vi "rsidr_core_global.vi"() -> ()   [LabVIEW 2020, in "Rohde&Schwarz CMWXP NR FR1 Measurement.lvlib"] (continued)
count for modulation measurements exceeding the specified modulation limits.\nDefault unit:  %\n\n<3_Ripple1>\n float\nMax (range 1) - min (range 1)\nDefault unit:  dB\n\n<4_Ripple2>\n float\nMax (range 2) - min (range 2)\nDefault unit:  dB\n\n<5_MaxR1MinR2>\n float\nMax (range 1) - min (range 2)\nDefault unit:  dB\n\n<6_MaxR2MinR1>\n float\nMax (range 2) - min (range 1)\nDefault unit:  dB\n\n<7_MinR1>\n float\nMin (range 1)\nDefault unit:  dB\n\n<8_MaxR1>\n float\nMax (range 1)\nDefault unit:  dB\n\n<9_MinR2>\n float\nMin (range 2)\nDefault unit:  dB\n\n<10_MaxR2>\n float\nMax (range 2)\nDefault unit:  dB\n\nAvailable Repeated Capabilities:\ninstance: i0, i1, i2, i3, i4, i5, i6, i7, i8, i9, i10, i11, i12, i13, i14, i15, i16, i17, i18, i19, i20, i21, i22, i23, i24, i25, i26, i27, i28, i29, i30, i31, i32\r\n\nRemote-control command(s):\nREAD:NRSub:MEAS<i>:MEValuation:ESFLatness:EXTReme?"}, {"Level"=4, "Class Only"=FALSE, "Identifier"="RSCMWXPNRFR1M_ATTR_READ_MULTI_EVAL_MEAS_ES_FLATNESS_STANDARD_DEVIATION_RESULTS", "Descriptive Name"="Read Multi Eval Meas ES Flatness Standard Deviation Results", "Data Type"=enum."RawString", "Command"="READ:NRS:MEAS{instance}:MEV:ESFL:SDEV?", "Access"=enum."Read Only", "Range Table"="", "Read Callback"="", "Write Callback"="", "Range Callback"="", "Check Callback"="", "Rngtable Callback"="", "Coerce Callback"="", "Supported Models"="", "Instrument Options"="", "Check Status Callback"="", "Flags"=0, "Help"="Return standard deviation single value results of the equalizer spectrum flatness measurement.\n\n<1_Reliability>\n decimal\n\n<2_OutOfTol>\n decimal\nOut of tolerance result, i.e. percentage of measurement intervals of the statistic count for modulation measurements exceeding the specified modulation limits.\nDefault unit:  %\n\n<3_Ripple1>\n float\nMax (range 1) - min (range 1)\nDefault unit:  dB\n\n<4_Ripple2>\n float\nMax (range 2) - min (range 2)\nDefault unit:  dB\n\n<5_MaxR1MinR2>\n float\nMax (range 1) - min (range 2)\nDefault unit:  dB\n\n<6_MaxR2MinR1>\n float\nMax (range 2) - min (range 1)\nDefault unit:  dB\n\n<7_MinR1>\n float\nMin (range 1)\nDefault unit:  dB\n\n<8_MaxR1>\n float\nMax (range 1)\nDefault unit:  dB\n\n<9_MinR2>\n float\nMin (range 2)\nDefault unit:  dB\n\n<10_MaxR2>\n float\nMax (range 2)\nDefault unit:  dB\n\nAvailable Repeated Capabilities:\ninstance: i0, i1, i2, i3, i4, i5, i6, i7, i8, i9, i10, i11, i12, i13, i14, i15, i16, i17, i18, i19, i20, i21, i22, i23, i24, i25, i26, i27, i28, i29, i30, i31, i32\r\n\nRemote-control command(s):\nREAD:NRSub:MEAS<i>:MEValuation:ESFLatness:SDEViation?"}, {"Level"=4, "Class Only"=FALSE, "Identifier"="RSCMWXPNRFR1M_ATTR_FETCH_MULTI_EVAL_MEAS_ES_FLATNESS_CURRENT_RESULTS", "Descriptive Name"="Fetch Multi Eval Meas ES Flatness Current Results", "Data Type"=enum."RawString", "Command"="FETC:NRS:MEAS{instance}:MEV:ESFL:CURR?", "Access"=enum."Read Only", "Range Table"="", "Read Callback"="", "Write Callback"="", "Range Callback"="", "Check Callback"="", "Rngtable Callback"="", "Coerce Callback"="", "Supported Models"="", "Instrument Options"="", "Check Status Callback"="", "Flags"=0, "Help"="Return current single value results of the equalizer spectrum flatness measurement.\n\n<1_Reliability>\n decimal\n\n<2_OutOfTol>\n decimal\nOut of tolerance result, i.e. percentage of measurement intervals of the statistic count for modulation measurements exceeding the specified modulation limits.\nDefault unit:  %\n\n<3_Ripple1>\n float\nMax (range 1) - min (range 1)\nDefault unit:  dB\n\n<4_Ripple2>\n float\nMax (range 2) - min (range 2)\nDefault unit:  dB\n\n<5_MaxR1MinR2>\n float\nMax (range 1) - min (range 2)\nDefault unit:  dB\n\n<6_MaxR2MinR1>\n float\nMax (range 2) - min (range 1)\nDefault unit:  dB\n\n<7_MinR1>\n float\nMin (range 1)\nDefault unit:  dB\n\n<8_MaxR1>\n float\nMax (range 1)\nDefault unit:  dB\n\n<9_MinR2>\n float\nMin (range 2)\nDefault unit:  dB\n\n<10_MaxR2>\n float\nMax (range 2)\nDefault unit:  dB\n\nAvailable Repeated Capabilities:\ninstance: i0, i1, i2, i3, i4, i5, i6, i7, i8, i9, i10, i11, i12, i13, i14, i15, i16, i17, i18, i19, i20, i21, i22, i23, i24, i25, i26, i27, i28, i29, i30, i31, i32\r\n\nRemote-control command(s):\nFETCh:NRSub:MEAS<i>:MEValuation:ESFLatness:CURRent?"}, {"Level"=4, "Class Only"=FALSE, "Identifier"="RSCMWXPNRFR1M_ATTR_FETCH_MULTI_EVAL_MEAS_ES_FLATNESS_AVERAGE_RESULTS", "Descriptive Name"="Fetch Multi Eval Meas ES Flatness Average Results", "Data Type"=enum."RawString", "Command"="FETC:NRS:MEAS{instance}:MEV:ESFL:AVER?", "Access"=enum."Read Only", "Range Table"="", "Read Callback"="", "Write Callback"="", "Range Callback"="", "Check Callback"="", "Rngtable Callback"="", "Coerce Callback"="", "Supported Models"="", "Instrument Options"="", "Check Status Callback"="", "Flags"=0, "Help"="Return average single value results of the equalizer spectrum flatness measurement.\n\n<1_Reliability>\n decimal\n\n<2_OutOfTol>\n decimal\nOut of tolerance result, i.e. percentage of measurement intervals of the statistic count for modulation measurements exceeding the specified modulation limits.\nDefault unit:  %\n\n<3_Ripple1>\n float\nMax (range 1) - min (range 1)\nDefault unit:  dB\n\n<4_Ripple2>\n float\nMax (range 2) - min (range 2)\nDefault unit:  dB\n\n<5_MaxR1MinR2>\n float\nMax (range 1) - min (range 2)\nDefault unit:  dB\n\n<6_MaxR2MinR1>\n float\nMax (range 2) - min (range 1)\nDefault unit:  dB\n\n<7_MinR1>\n float\nMin (range 1)\nDefault unit:  dB\n\n<8_MaxR1>\n float\nMax (range 1)\nDefault unit:  dB\n\n<9_MinR2>\n float\nMin (range 2)\nDefault unit:  dB\n\n<10_MaxR2>\n float\nMax (range 2)\nDefault unit:  dB\n\nAvailable Repeated Capabilities:\ninstance: i0, i1, i2, i3, i4, i5, i6, i7, i8, i9, i10, i11, i12, i13, i14, i15, i16, i17, i18, i19, i20, i21, i22, i23, i24, i25, i26, i27, i28, i29, i30, i31, i32\r\n\nRemote-control command(s):\nFETCh:NRSub:MEAS<i>:MEValuation:ESFLatness:AVERage?"}, {"Level"=4, "Class Only"=FALSE, "Identifier"="RSCMWXPNRFR1M_ATTR_FETCH_MULTI_EVAL_MEAS_ES_FLATNESS_EXTREME_RESULTS", "Descriptive Name"="Fetch Multi Eval Meas ES Flatness Extreme Results", "Data Type"=enum."RawString", "Command"="FETC:NRS:MEAS{instance}:MEV:ESFL:EXTR?", "Access"=enum."Read Only", "Range Table"="", "Read Callback"="", "Write Callback"="", "Range Callback"="", "Check Callback"="", "Rngtable Callback"="", "Coerce Callback"="", "Supported Models"="", "Instrument Options"="", "Check Status Callback"="", "Flags"=0, "Help"="Return extreme single value results of the equalizer spectrum flatness measurement.\n\n<1_Reliability>\n decimal\n\n<2_OutOfTol>\n decimal\nOut of tolerance result, i.e. percentage of measurement intervals of the statistic count for modulation measurements exceeding the specified modulation limits.\nDefault unit:  %\n\n<3_Ripple1>\n float\nMax (range 1) - min (range 1)\nDefault unit:  dB\n\n<4_Ripple2>\n float\nMax (range 2) - min (range 2)\nDefault unit:  dB\n\n<5_MaxR1MinR2>\n float\nMax (range 1) - min (range 2)\nDefault unit:  dB\n\n<6_MaxR2MinR1>\n float\nMax (range 2) - min (range 1)\nDefault unit:  dB\n\n<7_MinR1>\n float\nMin (range 1)\nDefault unit:  dB\n\n<8_MaxR1>\n float\nMax (range 1)\nDefault unit:  dB\n\n<9_MinR2>\n float\nMin (range 2)\nDefault unit:  dB\n\n<10_MaxR2>\n float\nMax (range 2)\nDefault unit:  dB\n\nAvailable Repeated Capabilities:\ninstance: i0, i1, i2, i3, i4, i5, i6, i7, i8, i9, i10, i11, i12, i13, i14, i15, i16, i17, i18, i19, i20, i21, i22, i23, i24, i25, i26, i27, i28, i29, i30, i31, i32\r\n\nRemote-control command(s):\nFETCh:NRSub:MEAS<i>:MEValuation:ESFLatness:EXTReme?"}, {"Level"=4, "Class Only"=FALSE, "Identifier"="RSCMWXPNRFR1M_ATTR_FETCH_MULTI_EVAL_MEAS_ES_FLATNESS_STANDARD_DEVIATION_RESULTS", "Descriptive Name"="Fetch Multi Eval Meas ES Flatness Standard Deviation Results", "Data Type"=enum."RawString", "Command"="FETC:NRS:MEAS{instance}:MEV:ESFL:SDEV?", "Access"=enum."Read Only", "Range Table"="", "Read Callback"="", "Write Callback"="", "Range Callback"="", "Check Callback"="", "Rngtable Callback"="", "Coerce Callback"="", "Supported Models"="", "Instrument Options"="", "Check Status Callback"="", "Flags"=0, "Help"="Return standard deviation single value results of the equalizer spectrum flatness measurement.\n\n<1_Reliability>\n decimal\n\n<2_OutOfTol>\n decimal\nOut of tolerance result, i.e. percentage of measurement intervals of the statistic count for modulation measurements exceeding the specified modulation limits.\nDefault unit:  %\n\n<3_Ripple1>\n float\nMax (range 1) - min (range 1)\nDefault unit:  dB\n\n<4_Ripple2>\n float\nMax (range 2) - min (range 2)\nDefault unit:  dB\n\n<5_MaxR1MinR2>\n float\nMax (range 1) - min (range 2)\nDefault unit:  dB\n\n<6_MaxR2MinR1>\n float\nMax (range 2) - min (range 1)\nDefault unit:  dB\n\n<7_MinR1>\n float\nMin (range 1)\nDefault unit:  dB\n\n<8_MaxR1>\n float\nMax (range 1)\nDefault unit:  dB\n\n<9_MinR2>\n float\nMin (range 2)\nDefault unit:  dB\n\n<10_MaxR2>\n float\nMax (range 2)\nDefault unit:  dB\n\nAvailable Repeated Capabilities:\ninstance: i0, i1, i2, i3, i4, i5, i6, i7, i8, i9, i10, i11, i12, i13, i14, i15, i16, i17, i18, i19, i20, i21, i22, i23, i24, i25, i26, i27, i28, i29, i30, i31, i32\r\n\nRemote-control command(s):\nFETCh:NRSub:MEAS<i>:MEValuation:ESFLatness:SDEViation?"}, {"Level"=4, "Class Only"=FALSE, "Identifier"="RSCMWXPNRFR1M_ATTR_QUERY_MULTI_EVAL_MEAS_ES_FLATNESS_CURRENT_LIMIT_CHECK_RESULTS", "Descriptive Name"="Query Multi Eval Meas ES Flatness Current Limit Check Results", "Data Type"=enum."RawString", "Command"="CALC:NRS:MEAS{instance}:MEV:ESFL:CURR?", "Access"=enum."Read Only", "Range Table"="", "Read Callback"="", "Write Callback"="", "Range Callback"="", "Check Callback"="", "Rngtable Callback"="", "Coerce Callback"="", "Supported Models"="", "Instrument Options"="", "Check Status Callback"="", "Flags"=0, "Help"="Return current limit check results for the equalizer spectrum flatness measurement.\n\nReturn values:\n<Reliability>\n decimal\n\n<OutOfTolerance>\n decimal\nOut of tolerance result, i.e. percentage of measurement intervals of the statistic count for modulation measurements exceeding the specified modulation limits.\nDefault unit:  %\n\n<Ripple1>\n Limit check result for max (range 1) - min (range 1)\n\n<Ripple2>\n Limit check result for max (range 2) - min (range 2)\n\n<MaxR1MinR2>\n Limit check result for max (range 1) - min (range 2)\n\n<MaxR2MinR1>\n Limit check result for max (range 2) - min (range 1)\n\nAvailable Repeated Capabilities:\ninstance: i0, i1, i2, i3, i4, i5, i6, i7, i8, i9, i10, i11, i12, i13, i14, i15, i16, i17, i18, i19, i20, i21, i22, i23, i24, i25, i26, i27, i28, i29, i30, i31, i32\r\n\nRemote-control command(s):\nCALCulate:NRSub:MEAS<i>:MEValuation:ESFLatness:CURRent?"}, {"Level"=4, "Class Only"=FALSE, "Identifier"="RSCMWXPNRFR1M_ATTR_QUERY_MULTI_EVAL_MEAS_ES_FLATNESS_AVERAGE_LIMIT_CHECK_RESULTS", "Descriptive Name"="Query Multi Eval Meas ES Flatness Average Limit Check Results", "Data Type"=enum."RawString", "Command"="CALC:NRS:MEAS{instance}:MEV:ESFL:AVER?", "Access"=enum."Read Only", "Range Table"="", "Read Callback"="", "Write Callback"="", "Range Callback"="", "Check Callback"="", "Rngtable Callback"="", "Coerce Callback"="", "Supported Models"="", "Instrument Options"="", "Check Status Callback"="", "Flags"=0, "Help"="Return average results for the equalizer spectrum flatness measurement.\n\nReturn values:\n<Reliability>\n decimal\n\n<OutOfTolerance>\n decimal\nOut of tolerance result, i.e. percentage of measurement intervals of the statistic count for modulation measurements exceeding the specified modulation limits.\nDefault unit:  %\n\n<Ripple1>\n Limit check result for max (range 1) - min (range 1)\n\n<Ripple2>\n Limit check result for max (range 2) - min (range 2)\n\n<MaxR1MinR2>\n Limit check result for max (range 1) - min (range 2)\n\n<MaxR2MinR1>\n Limit check result for max (range 2) - min (range 1)\n\nAvailable Repeated Capabilities:\ninstance: i0, i1, i2, i3, i4, i5, i6, i7, i8, i9, i10, i11, i12, i13, i14, i15, i16, i17, i18, i19, i20, i21, i22, i23, i24, i25, i26, i27, i28, i29, i30, i31, i32\r\n\nRemote-control command(s):\nCALCulate:NRSub:MEAS<i>:MEValuation:ESFLatness:AVERage?"}, {"Level"=4, "Class Only"=FALSE, "Identifier"="RSCMWXPNRFR1M_ATTR_QUERY_MULTI_EVAL_MEAS_ES_FLATNESS_EXTREME_LIMIT_CHECK_RESULTS", "Descriptive Name"="Query Multi Eval Meas ES Flatness Extreme Limit Check Results", "Data Type"=enum."RawString", "Command"="CALC:NRS:MEAS{instance}:MEV:ESFL:EXTR?", "Access"=enum."Read Only", "Range Table"="", "Read Callback"="", "Write Callback"="", "Range Callback"="", "Check Callback"="", "Rngtable Callback"="", "Coerce Callback"="", "Supported Models"="", "Instrument Options"="", "Check Status Callback"="", "Flags"=0, "Help"="Return extreme limit check results for the equalizer spectrum flatness measurement.\n\nReturn values:\n<Reliability>\n decimal\n\n<OutOfTolerance>\n decimal\nOut of tolerance result, i.e. percentage of measurement intervals of the statistic count for modulation measurements exceeding the specified modulation limits.\nDefault unit:  %\n\n<Ripple1>\n Limit check result for max (range 1) - min (range 1)\n\n<Ripple2>\n Limit check result for max (range 2) - min (range 2)\n\n<MaxR1MinR2>\n Limit check result for max (range 1) - min (range 2)\n\n<MaxR2MinR1>\n Limit check result for max (range 2) - min (range 1)\n\nAvailable Repeated Capabilities:\ninstance: i0, i1, i2, i3, i4, i5, i6, i7, i8, i9, i10, i11, i12, i13, i14, i15, i16, i17, i18, i19, i20, i21, i22, i23, i24, i25, i26, i27, i28, i29, i30, i31, i32\r\n\nRemote-control command(s):\nCALCulate:NRSub:MEAS<i>:MEValuation:ESFLatness:EXTReme?"}, {"Level"=4, "Class Only"=FALSE, "Identifier"="RSCMWXPNRFR1M_ATTR_FETCH_MULTI_EVAL_MEAS_ES_FLATNESS_SUBCARRIER_INDEX_RESULTS", "Descriptive Name"="Fetch Multi Eval Meas ES Flatness Subcarrier Index Results", "Data Type"=enum."RawString", "Command"="FETC:NRS:MEAS{instance}:MEV:ESFL:CURR:SCIN?", "Access"=enum."Read Only", "Range Table"="", "Read Callback"="", "Write Callback"="", "Range Callback"="", "Check Callback"="", "Rngtable Callback"="", "Coerce Callback"="", "Supported Models"="", "Instrument Options"="", "Check Status Callback"="", "Flags"=0, "Help"="Returns subcarrier indices of the equalizer spectrum flatness measurement. At these SC indices, the current minimum and maximum power of the equalizer coefficients have been detected within range 1 and range 2.\n\nReturn values:\n<Reliability>\n decimal\n\n<OutOfTolerance>\n decimal\nOut of tolerance result, i.e. percentage of measurement intervals of the statistic count for modulation measurements exceeding the specified modulation limits.\nDefault unit:  %\n\n<Maximum1>\n decimal\nSC index of 'Max (Range 1)'\n\n<Minimum1>\n decimal\nSC index of 'Min (Range 1)'\n\n<Maximum2>\n decimal\nSC index of 'Max (Range 2)'\n\n<Minimum2>\n decimal\nSC index of 'Min (Range 2)'\n\nAvailable Repeated Capabilities:\ninstance: i0, i1, i2, i3, i4, i5, i6, i7, i8, i9, i10, i11, i12, i13, i14, i15, i16, i17, i18, i19, i20, i21, i22, i23, i24, i25, i26, i27, i28, i29, i30, i31, i32\r\n\nRemote-control command(s):\nFETCh:NRSub:MEAS<i>:MEValuation:ESFLatness:CURRent:SCINdex?"}, {"Level"=3, "Class Only"=TRUE, "Identifier"="", "Descriptive Name"="Spectrum Emission Mask", "Data Type"=enum."ViInt32", "Command"="", "Access"=enum."Read Only", "Range Table"="", "Read Callback"="", "Write Callback"="", "Range Callback"="", "Check Callback"="", "Rngtable Callback"="", "Coerce Callback"="", "Supported Models"="", "Instrument Options"="", "Check Status Callback"="", "Flags"=0, "Help"="The commands in this class return the spectrum emission results."}, {"Level"=4, "Class Only"=FALSE, "Identifier"="RSCMWXPNRFR1M_ATTR_READ_MULTI_EVAL_MEAS_SEM_CURRENT_RESULTS", "Descriptive Name"="Read Multi Eval Meas SEM Current Results", "Data Type"=enum."RawString", "Command"="READ:NRS:MEAS{instance}:MEV:SEM:CURR?", "Access"=enum."Read Only", "Range Table"="", "Read Callback"="", "Write Callback"="", "Range Callback"="", "Check Callback"="", "Rngtable Callback"="", "Coerce Callback"="", "Supported Models"="", "Instrument Options"="", "Check Status Callback"="", "Flags"=0, "Help"="Return the current single value results of the spectrum emission measurement.\n\nReturn values:\n<Reliability>\n decimal\n\n<OutOfTolerance>\n decimal\nOut of tolerance result, i.e. percentage of measurement intervals of the statistic count for spectrum emission measurements exceeding the specified spectrum emission mask limits.\nDefault unit:  % \n\n<OBW>\n float\nOccupied bandwidth\nDefault unit:  Hz \n\n<TXpower>\n float\nTotal TX power in the slot\nDefault unit:  dBm\n\nAvailable Repeated Capabilities:\ninstance: i0, i1, i2, i3, i4, i5, i6, i7, i8, i9, i10, i11, i12, i13, i14, i15, i16, i17, i18, i19, i20, i21, i22, i23, i24, i25, i26, i27, i28, i29, i30, i31, i32\r\n\nRemote-control command(s):\nREAD:NRSub:MEAS<i>:MEValuation:SEMask:CURRent?"}, {"Level"=4, "Class Only"=FALSE, "Identifier"="RSCMWXPNRFR1M_ATTR_READ_MULTI_EVAL_MEAS_SEM_AVERAGE_RESULTS", "Descriptive Name"="Read Multi Eval Meas SEM Average Results", "Data Type"=enum."RawString", "Command"="READ:NRS:MEAS{instance}:MEV:SEM:AVER?", "Access"=enum."Read Only", "Range Table"="", "Read Callback"="", "Write Callback"="", "Range Callback"="", "Check Callback"="", "Rngtable Callback"="", "Coerce Callback"="", "Supported Models"="", "Instrument Options"="", "Check Status Callback"="", "Flags"=0, "Help"="Return the average single value results of the spectrum emission measurement.\n\nReturn values:\n<Reliability>\n decimal\n\n<OutOfTolerance>\n decimal\nOut of tolerance result, i.e. percentage of measurement intervals of the statistic count for spectrum emission measurements exceeding the specified spectrum emission mask limits.\nDefault unit:  % \n\n<OBW>\n float\nOccupied bandwidth\nDefault unit:  Hz \n\n<TXpower>\n float\nTotal TX power in the slot\nDefault unit:  dBm\n\nAvailable Repeated Capabilities:\ninstance: i0, i1, i2, i3, i4, i5, i6, i7, i8, i9, i10, i11, i12, i13, i14, i15, i16, i17, i18, i19, i20, i21, i22, i23, i24, i25, i26, i27, i28, i29, i30, i31, i32\r\n\nRemote-control command(s):\nREAD:NRSub:MEAS<i>:MEValuation:SEMask:AVERage?"}, {"Level"=4, "Class Only"=FALSE, "Identifier"="RSCMWXPNRFR1M_ATTR_READ_MULTI_EVAL_MEAS_SEM_STANDARD_DEVIATION_RESULTS", "Descriptive Name"="Read Multi Eval Meas SEM Standard Deviation Results", "Data Type"=enum."RawString", "Command"="READ:NRS:MEAS{instance}:MEV:SEM:SDEV?", "Access"=enum."Read Only", "Range Table"="", "Read Callback"="", "Write Callback"="", "Range Callback"="", "Check Callback"="", "Rngtable Callback"="", "Coerce Callback"="", "Supported Models"="", "Instrument Options"="", "Check Status Callback"="", "Flags"=0, "Help"="Return the standard deviation single value results of the spectrum emission measurement.\n\nReturn values:\n<Reliability>\n decimal\n\n<OutOfTolerance>\n decimal\nOut of tolerance result, i.e. percentage of measurement intervals of the statistic count for spectrum emission measurements exceeding the specified spectrum emission mask limits.\nDefault unit:  % \n\n<OBW>\n float\nOccupied bandwidth\nDefault unit:  Hz \n\n<TXpower>\n float\nTotal TX power in the slot\nDefault unit:  dBm\n\nAvailable Repeated Capabilities:\ninstance: i0, i1, i2, i3, i4, i5, i6, i7, i8, i9, i10, i11, i12, i13, i14, i15, i16, i17, i18, i19, i20, i21, i22, i23, i24, i25, i26, i27, i28, i29, i30, i31, i32\r\n\nRemote-control command(s):\nREAD:NRSub:MEAS<i>:MEValuation:SEMask:SDEViation?"}, {"Level"=4, "Class Only"=FALSE, "Identifier"="RSCMWXPNRFR1M_ATTR_FETCH_MULTI_EVAL_MEAS_SEM_CURRENT_RESULTS", "Descriptive Name"="Fetch Multi Eval Meas SEM Current Results", "Data Type"=enum."RawString", "Command"="FETC:NRS:MEAS{instance}:MEV:SEM:CURR?", "Access"=enum."Read Only", "Range Table"="", "Read Callback"="", "Write Callback"="", "Range Callback"="", "Check Callback"="", "Rngtable Callback"="", "Coerce Callback"="", "Supported Models"="", "Instrument Options"="", "Check Status Callback"="", "Flags"=0, "Help"="Return the current single value results of the spectrum emission measurement.\n\nReturn values:\n<Reliability>\n decimal\n\n<OutOfTolerance>\n decimal\nOut of tolerance result, i.e. percentage of measurement intervals of the statistic count for spectrum emission measurements exceeding the specified spectrum emission mask limits.\nDefault unit:  % \n\n<OBW>\n float\nOccupied bandwidth\nDefault unit:  Hz \n\n<TXpower>\n float\nTotal TX power in the slot\nDefault unit:  dBm\n\nAvailable Repeated Capabilities:\ninstance: i0, i1, i2, i3, i4, i5, i6, i7, i8, i9, i10, i11, i12, i13, i14, i15, i16, i17, i18, i19, i20, i21, i22, i23, i24, i25, i26, i27, i28, i29, i30, i31, i32\r\n\nRemote-control command(s):\nFETCh:NRSub:MEAS<i>:MEValuation:SEMask:CURRent?"}, {"Level"=4, "Class Only"=FALSE, "Identifier"="RSCMWXPNRFR1M_ATTR_FETCH_MULTI_EVAL_MEAS_SEM_AVERAGE_RESULTS", "Descriptive Name"="Fetch Multi Eval Meas SEM Average Results", "Data Type"=enum."RawString", "Command"="FETC:NRS:MEAS{instance}:MEV:SEM:AVER?", "Access"=enum."Read Only", "Range Table"="", "Read Callback"="", "Write Callback"="", "Range Callback"="", "Check Callback"="", "Rngtable Callback"="", "Coerce Callback"="", "Supported Models"="", "Instrument Options"="", "Check Status Callback"="", "Flags"=0, "Help"="Return the average single value results of the spectrum emission measurement.\n\nReturn values:\n<Reliability>\n decimal\n\n<OutOfTolerance>\n decimal\nOut of tolerance result, i.e. percentage of measurement intervals of the statistic count for spectrum emission measurements exceeding the specified spectrum emission mask limits.\nDefault unit:  % \n\n<OBW>\n float\nOccupied bandwidth\nDefault unit:  Hz \n\n<TXpower>\n float\nTotal TX power in the slot\nDefault unit:  dBm\n\nAvailable Repeated Capabilities:\ninstance: i0, i1, i2, i3, i4, i5, i6, i7, i8, i9, i10, i11, i12, i13, i14, i15, i16, i17, i18, i19, i20, i21, i22, i23, i24, i25, i26, i27, i28, i29, i30, i31, i32\r\n\nRemote-control command(s):\nFETCh:NRSub:MEAS<i>:MEValuation:SEMask:AVERage?"}, {"Level"=4, "Class Only"=FALSE, "Identifier"="RSCMWXPNRFR1M_ATTR_FETCH_MULTI_EVAL_MEAS_SEM_STANDARD_DEVIATION_RESULTS", "Descriptive Name"="Fetch Multi Eval Meas SEM Standard Deviation Results", "Data Type"=enum."RawString", "Command"="FETC:NRS:MEAS{instance}:MEV:SEM:SDEV?", "Access"=enum."Read Only", "Range Table"="", "Read Callback"="", "Write Callback"="", "Range Callback"="", "Check Callback"="", "Rngtable Callback"="", "Coerce Callback"="", "Supported Models"="", "Instrument Options"="", "Check Status Callback"="", "Flags"=0, "Help"="Return the standard deviation single value results of the spectrum emission measurement.\n\nReturn values:\n<Reliability>\n decimal\n\n<OutOfTolerance>\n decimal\nOut of tolerance result, i.e. percentage of measurement intervals of the statistic count for spectrum emission measurements exceeding the specified spectrum emission mask limits.\nDefault unit:  % \n\n<OBW>\n float\nOccupied bandwidth\nDefault unit:  Hz \n\n<TXpower>\n float\nTotal TX power in the slot\nDefault unit:  dBm\n\nAvailable Repeated Capabilities:\ninstance: i0, i1, i2, i3, i4, i5, i6, i7, i8, i9, i10, i11, i12, i13, i14, i15, i16, i17, i18, i19, i20, i21, i22, i23, i24, i25, i26, i27, i28, i29, i30, i31, i32\r\n\nRemote-control command(s):\nFETCh:NRSub:MEAS<i>:MEValuation:SEMask:SDEViation?"}, {"Level"=4, "Class Only"=FALSE, "Identifier"="RSCMWXPNRFR1M_ATTR_QUERY_MULTI_EVAL_MEAS_SEM_CURRENT_LIMIT_CHECK_RESULTS", "Descriptive Name"="Query Multi Eval Meas SEM Current Limit Check Results", "Data Type"=enum."RawString", "Command"="CALC:NRS:MEAS{instance}:MEV:SEM:CURR?", "Access"=enum."Read Only", "Range Table"="", "Read Callback"="", "Write Callback"="", "Range Callback"="", "Check Callback"="", "Rngtable Callback"="", "Coerce Callback"="", "Supported Models"="", "Instrument Options"="", "Check Status Callback"="", "Flags"=0, "Help"="Return the current single value limit check results of the spectrum emission measurement.\n\nReturn values:\n<Reliability>\n decimal\n\n<OutOfTolerance>\n decimal\nOut of tolerance result, i.e. percentage of measurement intervals of the statistic count for spectrum emission measurements exceeding the specified spectrum emission mask limits.\nDefault unit:  % \n\n<OBWLimCheck>\n limit check result\n\n<TXpowerLimCheck>\n limit check result\n\nAvailable Repeated Capabilities:\ninstance: i0, i1, i2, i3, i4, i5, i6, i7, i8, i9, i10, i11, i12, i13, i14, i15, i16, i17, i18, i19, i20, i21, i22, i23, i24, i25, i26, i27, i28, i29, i30, i31, i32\r\n\nRemote-control command(s):\nCALCulate:NRSub:MEAS<i>:MEValuation:SEMask:CURRent?"}, {"Level"=4, "Class Only"=FALSE, "Identifier"="RSCMWXPNRFR1M_ATTR_QUERY_MULTI_EVAL_MEAS_SEM_AVERAGE_LIMIT_CHECK_RESULTS", "Descriptive Name"="Query Multi Eval Meas SEM Average Limit Check Results", "Data Type"=enum."RawString", "Command"="CALC:NRS:MEAS{instance}:MEV:SEM:AVER?", "Access"=enum."Read Only", "Range Table"="", "Read Callback"="", "Write Callback"="", "Range Callback"="", "Check Callback"="", "Rngtable Callback"="", "Coerce Callback"="", "Supported Models"="", "Instrument Options"="", "Check Status Callback"="", "Flags"=0, "Help"="Return the average single value limit check results of the spectrum emission measurement.\n\nReturn values:\n<Reliability>\n decimal\n\n<OutOfTolerance>\n decimal\nOut of tolerance result, i.e. percentage of measurement intervals of the statistic count for spectrum emission measurements exceeding the specified spectrum emission mask limits.\nDefault unit:  % \n\n<OBWLimCheck>\n limit check result\n\n<TXpowerLimCheck>\n limit check result\n\nAvailable Repeated Capabilities:\ninstance: i0, i1, i2, i3, i4, i5, i6, i7, i8, i9, i10, i11, i12, i13, i14, i15, i16, i17, i18, i19, i20, i21, i22, i23, i24, i25, i26, i27, i28, i29, i30, i31, i32\r\n\nRemote-control command(s):\nCALCulate:NRSub:MEAS<i>:MEValuation:SEMask:AVERage?"}, {"Level"=4, "Class Only"=FALSE, "Identifier"="RSCMWXPNRFR1M_ATTR_READ_MULTI_EVAL_MEAS_SEM_EXTREME_RESULTS", "Descriptive Name"="Read Multi Eval Meas SEM Extreme Results", "Data Type"=enum."RawString", "Command"="READ:NRS:MEAS{instance}:MEV:SEM:EXTR?", "Access"=enum."Read Only", "Range Table"="", "Read Callback"="", "Write Callback"="", "Range Callback"="", "Check Callback"="", "Rngtable Callback"="", "Coerce Callback"="", "Supported Models"="", "Instrument Options"="", "Check Status Callback"="", "Flags"=0, "Help"="Return the extreme single value results of the spectrum emission measurement.\n\nReturn values:  \n<Reliability>\n decimal\n\n<OutOfTolerance>\n decimal\nOut of tolerance result, i.e. percentage of measurement intervals of the statistic count for spectrum emission measurements exceeding the specified spectrum emission mask limits.\nDefault unit:  % \n\n<OBW>\n float\nOccupied bandwidth\nDefault unit:  Hz \n\n<TXpowerMin>\n float\nMinimum total TX power in the slot\nDefault unit:  dBm \n\n<TXpowerMax>\n float\nMaximum total TX power in the slot\nDefault unit:  dBm\n\nAvailable Repeated Capabilities:\ninstance: i0, i1, i2, i3, i4, i5, i6, i7, i8, i9, i10, i11, i12, i13, i14, i15, i16, i17, i18, i19, i20, i21, i22, i23, i24, i25, i26, i27, i28, i29, i30, i31, i32\r\n\nRemote-control command(s):\nREAD:NRSub:MEAS<i>:MEValuation:SEMask:EXTReme?"}, {"Level"=4, "Class Only"=FALSE, "Identifier"="RSCMWXPNRFR1M_ATTR_FETCH_MULTI_EVAL_MEAS_SEM_EXTREME_RESULTS", "Descriptive Name"="Fetch Multi Eval Meas SEM Extreme Results", "Data Type"=enum."RawString", "Command"="FETC:NRS:MEAS{instance}:MEV:SEM:EXTR?", "Access"=enum."Read Only", "Range Table"="", "Read Callback"="", "Write Callback"="", "Range Callback"="", "Check Callback"="", "Rngtable Callback"="", "Coerce Callback"="", "Supported Models"="", "Instrument Options"="", "Check Status Callback"="", "Flags"=0, "Help"="Return the extreme single value results of the spectrum emission measurement.\n\nReturn values:  \n<Reliability>\n decimal\n\n<OutOfTolerance>\n decimal\nOut of tolerance result, i.e. percentage of measurement intervals of the statistic count for spectrum emission measurements exceeding the specified spectrum emission mask limits.\nDefault unit:  % \n\n<OBW>\n float\nOccupied bandwidth\nDefault unit:  Hz \n\n<TXpowerMin>\n float\nMinimum total TX power in the slot\nDefault unit:  dBm \n\n<TXpowerMax>\n float\nMaximum total TX power in the slot\nDefault unit:  dBm\n\nAvailable Repeated Capabilities:\ninstance: i0, i1, i2, i3, i4, i5, i6, i7, i8, i9, i10, i11, i12, i13, i14, i15, i16, i17, i18, i19, i20, i21, i22, i23, i24, i25, i26, i27, i28, i29, i30, i31, i32\r\n\nRemote-control command(s):\nFETCh:NRSub:MEAS<i>:MEValuation:SEMask:EXTReme?"}, {"Level"=4, "Class Only"=FALSE, "Identifier"="RSCMWXPNRFR1M_ATTR_QUERY_MULTI_EVAL_MEAS_SEM_EXTREME_LIMIT_CHECK_RESULTS", "Descriptive Name"="Query Multi Eval Meas SEM Extreme Limit Check Results", "Data Type"=enum."RawString", "Command"="CALC:NRS:MEAS{instance}:MEV:SEM:EXTR?", "Access"=enum."Read Only", "Range Table"="", "Read Callback"="", "Write Callback"="", "Range Callback"="", "Check Callback"="", "Rngtable Callback"="", "Coerce Callback"="", "Supported Models"="", "Instrument Options"="", "Check Status Callback"="", "Flags"=0, "Help"="Return the extreme single value limit check results of the spectrum emission measurement.\n\nReturn values:  \n<Reliability>\n decimal\n\n<OutOfTolerance>\n decimal\nOut of tolerance result, i.e. percentage of measurement intervals of the statistic count for spectrum emission measurements exceeding the specified spectrum emission mask limits.\nDefault unit:  % \n\n<OBWLimCheck>\n limit check result\n\n<TXpowerMinLimCheck>\n limit check result\n\n<TXpowerMaxLimCheck>\n limit check result\n\nAvailable Repeated Capabilities:\ninstance: i0, i1, i2, i3, i4, i5, i6, i7, i8, i9, i10, i11, i12, i13, i14, i15, i16, i17, i18, i19, i20, i21, i22, i23, i24, i25, i26, i27, i28, i29, i30, i31, i32\r\n\nRemote-control command(s):\nCALCulate:NRSub:MEAS<i>:MEValuation:SEMask:EXTReme?"}, {"Level"=4, "Class Only"=FALSE, "Identifier"="RSCMWXPNRFR1M_ATTR_FETCH_MULTI_EVAL_MEAS_SEM_MARGIN_POSITIVE_CURRENT_RESULTS", "Descriptive Name"="Fetch Multi Eval Meas SEM Margin Positive Current Results", "Data Type"=enum."RawString", "Command"="FETC:NRS:MEAS{instance}:MEV:SEM:MARG:CURR:POS?", "Access"=enum."Read Only", "Range Table"="", "Read Callback"="", "Write Callback"="", "Range Callback"="", "Check Callback"="", "Rngtable Callback"="", "Coerce Callback"="", "Supported Models"="", "Instrument Options"="", "Check Status Callback"="", "Flags"=0, "Help"="Returns current spectrum emission mask margin results. A negative margin indicates that the trace is located above the limit line, i.e. the limit is exceeded. For each trace, the X and Y values of the margins for emission mask areas 1 to 12 are provided for positive offset frequencies. For inactive areas, NCAP is returned.\nReturned sequence: <Reliability>, <OutOfTolerance>, {<MarginX>, <MarginY>}area1, {...}area2, ..., {...}area12\n\nReturn values:  \n<Reliability>\n decimal\n\n<OutOfTolerance>\n decimal\nOut of tolerance result, i.e. percentage of measurement intervals of the statistic count for spectrum emission measurements exceeding the specified spectrum emission mask limits.\nDefault unit:  % \n\n<MarginX>\n float\nX-position of the margin of an area\nDefault unit:  Hz \n\n<MarginY>\n float\nY-value of the margin of an area\nDefault unit:  dB\n\nAvailable Repeated Capabilities:\ninstance: i0, i1, i2, i3, i4, i5, i6, i7, i8, i9, i10, i11, i12, i13, i14, i15, i16, i17, i18, i19, i20, i21, i22, i23, i24, i25, i26, i27, i28, i29, i30, i31, i32\r\n\nRemote-control command(s):\nFETCh:NRSub:MEAS<i>:MEValuation:SEMask:MARGin:CURRent:POSitiv?"}, {"Level"=4, "Class Only"=FALSE, "Identifier"="RSCMWXPNRFR1M_ATTR_FETCH_MULTI_EVAL_MEAS_SEM_MARGIN_POSITIVE_AVERAGE_RESULTS", "Descriptive Name"="Fetch Multi Eval Meas SEM Margin Positive Average Results", "Data Type"=enum."RawString", "Command"="FETC:NRS:MEAS{instance}:MEV:SEM:MARG:AVER:POS?", "Access"=enum."Read Only", "Range Table"="", "Read Callback"="", "Write Callback"="", "Range Callback"="", "Check Callback"="", "Rngtable Callback"="", "Coerce Callback"="", "Supported Models"="", "Instrument Options"="", "Check Status Callback"="", "Flags"=0, "Help"="Returns average spectrum emission mask margin results. A negative margin indicates that the trace is located above the limit line, i.e. the limit is exceeded. For each trace, the X and Y values of the margins for emission mask areas 1 to 12 are provided for positive offset frequencies. For inactive areas, NCAP is returned.\nReturned sequence: <Reliability>, <OutOfTolerance>, {<MarginX>, <MarginY>}area1, {...}area2, ..., {...}area12\n\nReturn values:  \n<Reliability>\n decimal\n\n<OutOfTolerance>\n decimal\nOut of tolerance result, i.e. percentage of measurement intervals of the statistic count for spectrum emission measurements exceeding the specified spectrum emission mask limits.\nDefault unit:  % \n\n<MarginX>\n float\nX-position of the margin of an area\nDefault unit:  Hz \n\n<MarginY>\n float\nY-value of the margin of an area\nDefault unit:  dB\n\nAvailable Repeated Capabilities:\ninstance: i0, i1, i2, i3, i4, i5, i6, i7, i8, i9, i10, i11, i12, i13, i14, i15, i16, i17, i18, i19, i20, i21, i22, i23, i24, i25, i26, i27, i28, i29, i30, i31, i32\r\n\nRemote-control command(s):\nFETCh:NRSub:MEAS<i>:MEValuation:SEMask:MARGin:AVERage:POSitiv?"}, {"Level"=4, "Class Only"=FALSE, "Identifier"="RSCMWXPNRFR1M_ATTR_FETCH_MULTI_EVAL_MEAS_SEM_MARGIN_POSITIVE_MINIMUM_RESULTS", "Descriptive Name"="Fetch Multi Eval Meas SEM Margin Positive Minimum Results", "Data Type"=enum."RawString", "Command"="FETC:NRS:MEAS{instance}:MEV:SEM:MARG:MIN:POS?", "Access"=enum."Read Only", "Range Table"="", "Read Callback"="", "Write Callback"="", "Range Callback"="", "Check Callback"="", "Rngtable Callback"="", "Coerce Callback"="", "Supported Models"="", "Instrument Options"="", "Check Status Callback"="", "Flags"=0, "Help"="Returns minimum spectrum emission mask margin results (i.e., results for the maximum traces). A negative margin indicates that the trace is located above the limit line, i.e. the limit is exceeded. For each trace, the X and Y values of the margins for emission mask areas 1 to 12 are provided for positive offset frequencies. For inactive areas, NCAP is returned.\nReturned sequence: <Reliability>, <OutOfTolerance>, {<MarginX>, <MarginY>}area1, {...}area2, ..., {...}area12\n\nReturn values:  \n<Reliability>\n decimal\n\n<OutOfTolerance>\n decimal\nOut of tolerance result, i.e. percentage of measurement intervals of the statistic count for spectrum emission measurements exceeding the specified spectrum emission mask limits.\nDefault unit:  % \n\n<MarginX>\n float\nX-position of the margin of an area\nDefault unit:  Hz \n\n<MarginY>\n float\nY-value of the margin of an area\nDefault unit:  dB\n\nAvailable Repeated Capabilities:\ninstance: i0, i1, i2, i3, i4, i5, i6, i7, i8, i9, i10, i11, i12, i13, i14, i15, i16, i17, i18, i19, i20, i21, i22, i23, i24, i25, i26, i27, i28, i29, i30, i31, i32\r\n\nRemote-control command(s):\nFETCh:NRSub:MEAS<i>:MEValuation:SEMask:MARGin:MINimum:POSitiv?"}, {"Level"=4, "Class Only"=FALSE, "Identifier"="RSCMWXPNRFR1M_ATTR_FETCH_MULTI_EVAL_MEAS_SEM_MARGIN_NEGATIVE_CURRENT_RESULTS", "Descriptive Name"="Fetch Multi Eval Meas SEM Margin Negative Current Results", "Data Type"=enum."RawString", "Command"="FETC:NRS:MEAS{instance}:MEV:SEM:MARG:CURR:NEG?", "Access"=enum."Read Only", "Range Table"="", "Read Callback"="", "Write Callback"="", "Range Callback"="", "Check Callback"="", "Rngtable Callback"="", "Coerce Callback"="", "Supported Models"="", "Instrument Options"="", "Check Status Callback"="", "Flags"=0, "Help"="Returns current spectrum emission mask margin results. A negative margin indicates that the trace is located above the limit line, i.e. the limit is exceeded. For each trace, the X and Y values of the margins for emission mask areas 1 to 12 are provided for negative offset frequencies. For inactive areas, NCAP is returned.\nReturned sequence: <Reliability>, <OutOfTolerance>, {<MarginX>, <MarginY>}area1, {...}area2, ..., {...}area12\n\nReturn values:  \n<Reliability>\n decimal\n\n<OutOfTolerance>\n decimal\nOut of tolerance result, i.e. percentage of measurement intervals of the statistic count for spectrum emission measurements exceeding the specified spectrum emission mask limits.\nDefault unit:  % \n\n<MarginX>\n float\nX-position of the margin of an area\nDefault unit:  Hz \n\n<MarginY>\n float\nY-value of the margin of an area\nDefault unit:  dB\n\nAvailable Repeated Capabilities:\ninstance: i0, i1, i2, i3, i4, i5, i6, i7, i8, i9, i10, i11, i12, i13, i14, i15, i16, i17, i18, i19, i20, i21, i22, i23, i24, i25, i26, i27, i28, i29, i30, i31, i32\r\n\nRemote-control command(s):\nFETCh:NRSub:MEAS<i>:MEValuation:SEMask:MARGin:CURRent:NEGativ?"}, {"Level"=4, "Class Only"=FALSE, "Identifier"="RSCMWXPNRFR1M_ATTR_FETCH_MULTI_EVAL_MEAS_SEM_MARGIN_NEGATIVE_AVERAGE_RESULTS", "Descriptive Name"="Fetch Multi Eval Meas SEM Margin Negative Average Results", "Data Type"=enum."RawString", "Command"="FETC:NRS:MEAS{instance}:MEV:SEM:MARG:AVER:NEG?", "Access"=enum."Read Only", "Range Table"="", "Read Callback"="", "Write Callback"="", "Range Callback"="", "Check Callback"="", "Rngtable Callback"="", "Coerce Callback"="", "Supported Models"="", "Instrument Options"="", "Check Status Callback"="", "Flags"=0, "Help"="Returns average spectrum emission mask margin results. A negative margin indicates that the trace is located above the limit line, i.e. the limit is exceeded. For each trace, the X and Y values of the margins for emission mask areas 1 to 12 are provided for negative offset frequencies. For inactive areas, NCAP is returned.\nReturned sequence: <Reliability>, <OutOfTolerance>, {<MarginX>, <MarginY>}area1, {...}area2, ..., {...}area12\n\nReturn values:  \n<Reliability>\n decimal\n\n<OutOfTolerance>\n decimal\nOut of tolerance result, i.e. percentage of measurement intervals of the statistic count for spectrum emission measurements exceeding the specified spectrum emission mask limits.\nDefault unit:  % \n\n<MarginX>\n float\nX-position of the margin of an area\nDefault unit:  Hz \n\n<MarginY>\n float\nY-value of the margin of an area\nDefault unit:  dB\n\nAvailable Repeated Capabilities:\ninstance: i0, i1, i2, i3, i4, i5, i6, i7, i8, i9, i10, i11, i12, i13, i14, i15, i16, i17, i18, i19, i20, i21, i22, i23, i24, i25, i26, i27, i28, i29, i30, i31, i32\r\n\nRemote-control command(s):\nFETCh:NRSub:MEAS<i>:MEValuation:SEMask:MARGin:AVERage:NEGativ?"}, {"Level"=4, "Class Only"=FALSE, "Identifier"="RSCMWXPNRFR1M_ATTR_FETCH_MULTI_EVAL_MEAS_SEM_MARGIN_NEGATIVE_MINIMUM_RESULTS", "Descriptive Name"="Fetch Multi Eval Meas SEM Margin Negative Minimum Results", "Data Type"=enum."RawString", "Command"="FETC:NRS:MEAS{instance}:MEV:SEM:MARG:MIN:NEG?", "Access"=enum."Read Only", "Range Table"="", "Read Callback"="", "Write Callback"="", "Range Callback"="", "Check Callback"="", "Rngtable Callback"="", "Coerce Callback"="", "Supported Models"="", "Instrument Options"="", "Check Status Callback"="", "Flags"=0, "Help"="Returns minimum spectrum emission mask margin results (i.e., results for the maximum traces). A negative margin indicates that the trace is located above the limit line, i.e. the limit is exceeded. For each trace, the X and Y values of the margins for emission mask areas 1 to 12 are provided for negative offset frequencies. For inactive areas, NCAP is returned.\nReturned sequence: <Reliability>, <OutOfTolerance>, {<MarginX>, <MarginY>}area1, {...}area2, ..., {...}area12\n\nReturn values:  \n<Reliability>\n decimal\n\n<OutOfTolerance>\n decimal\nOut of tolerance result, i.e. percentage of measurement intervals of the statistic count for spectrum 
